vi "Tiling second try.vi"() -> ()   [LabVIEW 2020]
uses:
  <vilib>/DAQmx/write.llb/DAQmx Write (Analog 1D Wfm NChan NSamp).vi
  <vilib>/DAQmx/create/channels.llb/DAQmx Create Channel (AO-Voltage-Basic).vi
  <vilib>/DAQmx/configure/timing.llb/DAQmx Timing (Use Waveform).vi
  <vilib>/DAQmx/miscellaneous.llb/DAQmx Fill In Error Info.vi
  <vilib>/measure/NI_MABase.lvlib
panel:
  out "Y Position 4":dbl=3.1101367187499998
  in  "OK Button":bool
  in  "Sawtooth Amplitude":dbl=0.23 format="%.2p"
  in  "Sawtooth Phase":dbl=180.0 format="%.2p"
  in  "Stop Analog Signal":bool
  out "# Samples written per channel":u32=1000
  in  "Exposure time (ms)":dbl=1000.0
  in  "Camera trigger delay (degrees)":dbl=-10.0 format="%.2p"
  in  "Sawtooth Offset":dbl=0.008 format="%.2p"
  out "Waveform Graph":waveform(dbl)[](graph)=[{"t0"=timestamp(0 s since 1904-01-01), "dt"=0.001, "Y"=array[1000 elements]}, {"t0"=timestamp(0 s since 1904-01-01), "dt"=0.001, "Y"=array[1000 elements]}, {"t0"=timestamp(0 s since 1904-01-01), "dt"=0.001, "Y"=array[1000 elements]}]
  in  "Z step size (um)":dbl=-0.2
  out "Number of Slices":dbl=100.0
  in  "Input will be multiplied by 5":dbl=20.0
  out "Error out":errorcluster
  in  "Close Communication":bool
  out "Z Position":dbl=3.559384999999838
  out "GetFirmwareVersion 2":string="3.03\r"
  out "Connected":bool=TRUE
  in  "SPIIPLUSCOM660Lib.IAsyncChannel":refnum<k7>
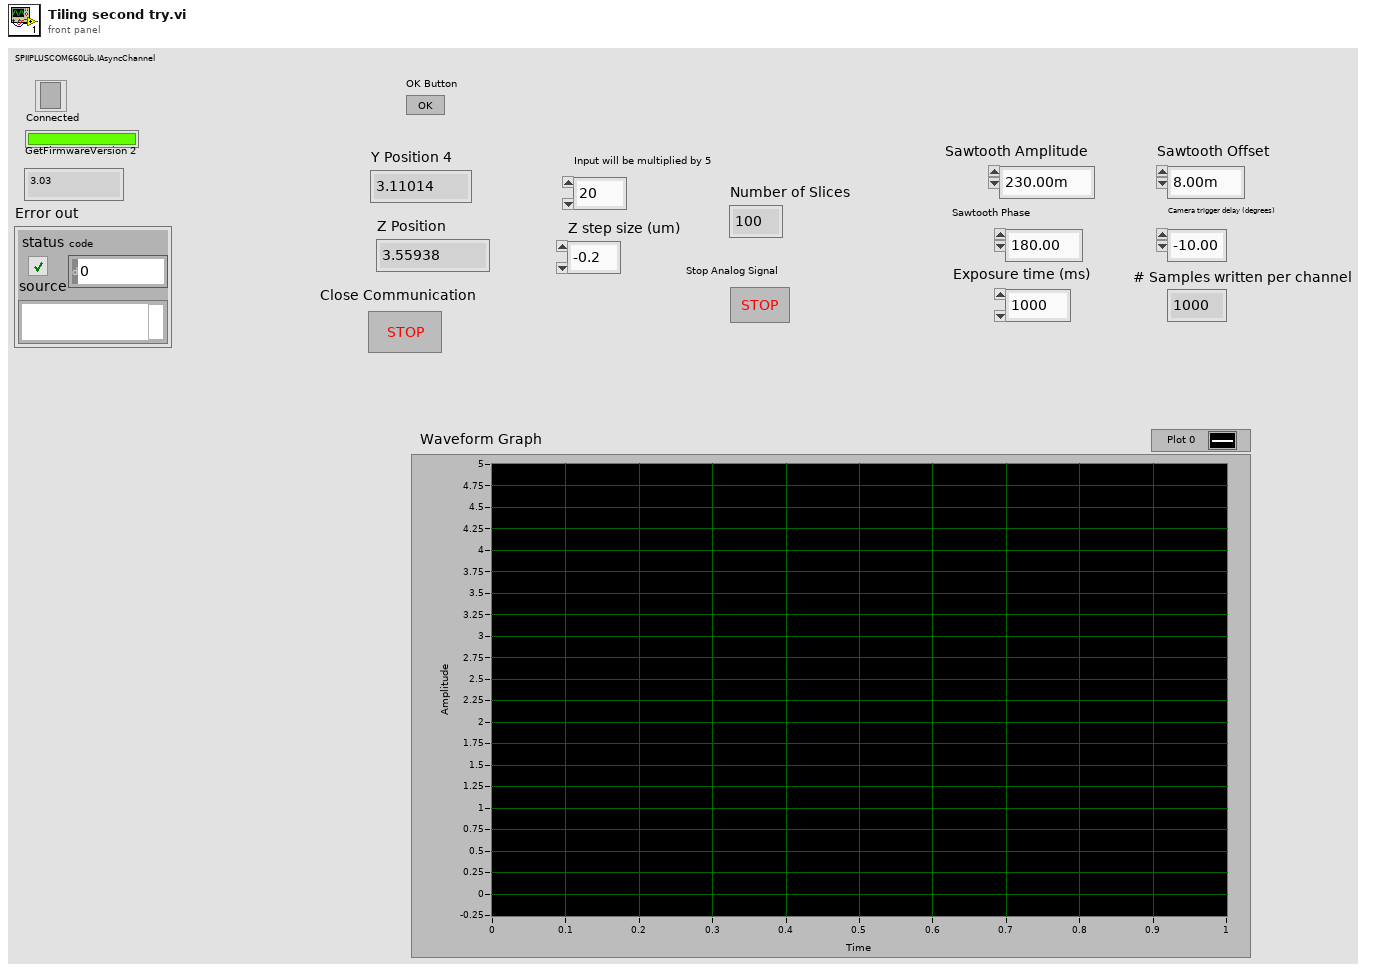
[diagram p1: front panel]
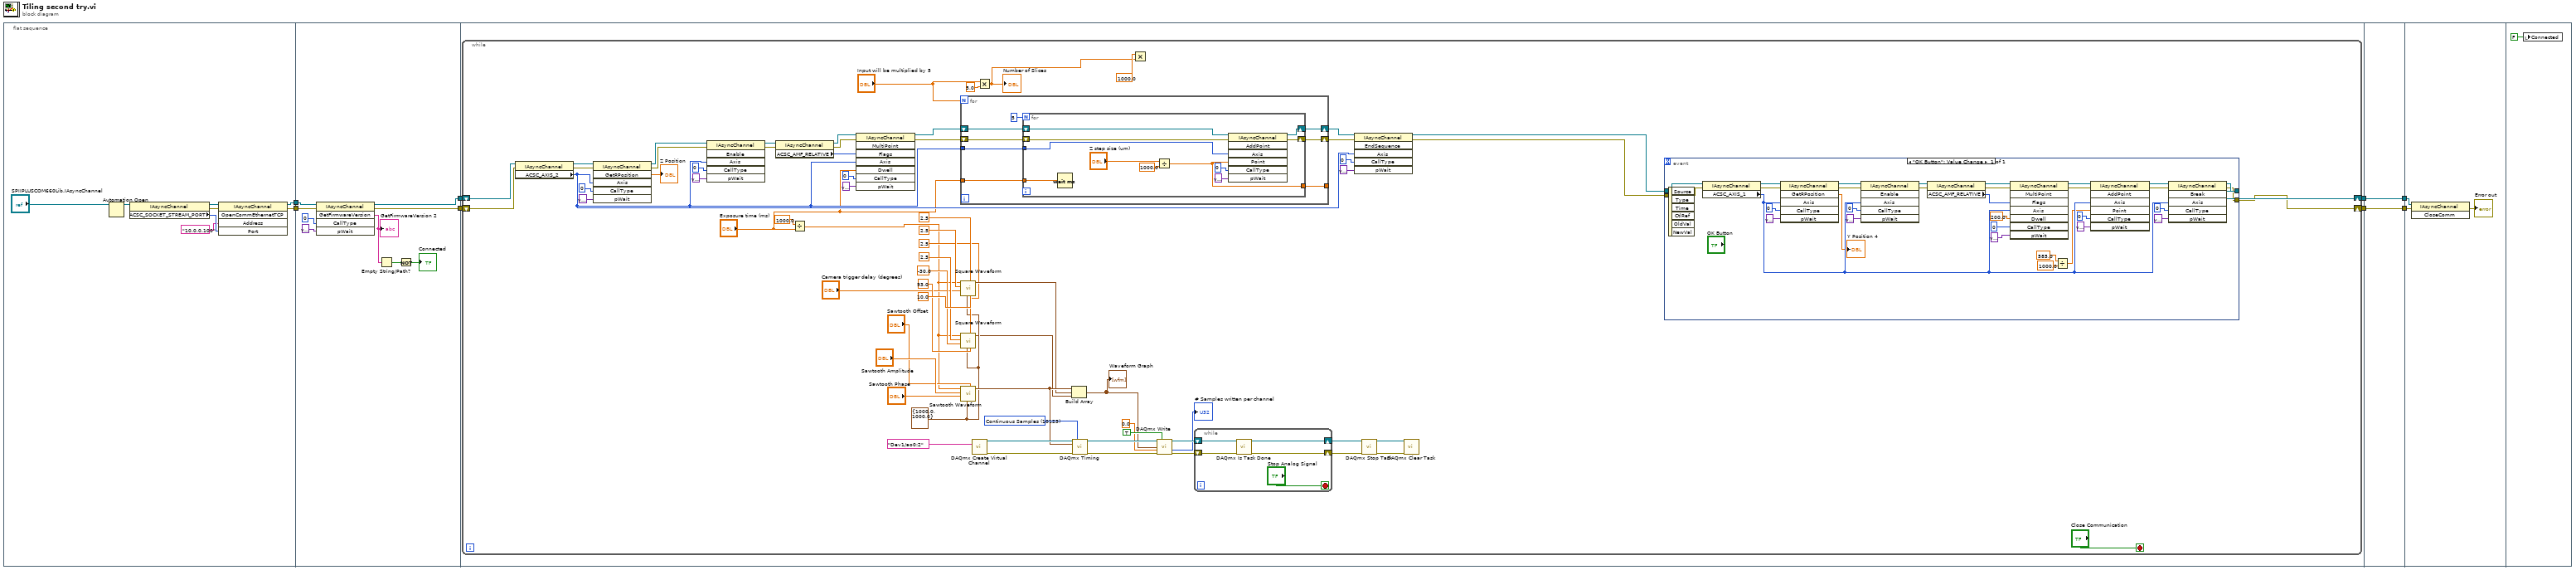
[diagram p0: block diagram]
diagram:
  n1 = flat-sequence {
    tunnel: [w11] -> w8
    tunnel: [w10] -> w7
    tunnel: w8 -> [w21]
    tunnel: w7 -> [w20]
    tunnel: [w18] -> w6
    tunnel: [w17] -> w5
    tunnel: w6 -> [w26]
    tunnel: w5 -> [w29]
    tunnel: [w28] -> w4
    tunnel: [w27] -> w3
    tunnel: w4 -> [w156]
    tunnel: w3 -> [w155]
    tunnel: [w156] -> w2
    tunnel: [w155] -> w1
    tunnel: w2 -> [w158]
    tunnel: w1 -> [w157]
    frame #0 {
      n2 = Automation Open(Automation Refnum="SPIIPLUSCOM660Lib.IAsyncChannel") -> (Automation Refnum=w16:refnum<k7>)  [unwired: 3 in, 1 out]
      n3 = property class="IAsyncChannel"(reference=w16) -> (reference out=w15:refnum<k7>, error out=w9:errorcluster, "ACSC_SOCKET_STREAM_PORT"=w13:i32)  [unwired: 1 in]
      n4 = invoke class="IAsyncChannel" method="OpenCommEthernetTCP"(reference=w15, error in=w9, "Address"="10.0.0.100", "Port"=w13) -> (reference out=w11:refnum<k7>, error out=w10:errorcluster)  [unwired: 1 in, 3 out]
    }
    frame #1 {
      n5 = invoke class="IAsyncChannel" method="GetFirmwareVersion"(reference=w21, error in=w20, "CallType"=u64 0, "pWait"=variant) -> (reference out=w18:refnum<k7>, error out=w17:errorcluster, "GetFirmwareVersion"=w23:string)  [unwired: 1 in, 2 out]
      "GetFirmwareVersion 2" <- w23
      n6 = Empty String/Path?(string/path=w23) -> (empty?=w22:bool)
      n7 = Not(x=w22) -> (.not. x?=→"Connected":bool)
    }
    frame #2 {
      n8 = while {
        shift-right: [w92] -> w28
        shift-left: w26 -> [w96]
        shift-right: [w91] -> w27
        shift-left: w29 -> [w95]
        stop <- "Close Communication" stop-if-true
        w54 = cluster{"Fs":dbl, "#s":dbl} {"Fs"=1000.0, "#s"=1000.0} ("sampling info")
        w77 = 10123 items=["Finite Samples"=10178, "Continuous Samples"=10123, "Hardware Timed Single Point"=12522] ("sample mode")
        n9 = property class="IAsyncChannel"(reference=w96, error in=w95) -> (reference out=w88:refnum<k7>, error out=w87:errorcluster, "ACSC_AXIS_2"=w90:i32)
        n10 = invoke class="IAsyncChannel" method="GetRPosition"(reference=w88, error in=w87, "Axis"=w90, "CallType"=u64 0, "pWait"=variant) -> (reference out=w36:refnum<k7>, error out=w34:errorcluster, "GetRPosition"=→"Z Position":dbl)  [unwired: 1 in, 3 out]
        n11 = invoke class="IAsyncChannel" method="Enable"(reference=w36, error in=w34, "Axis"=w90, "CallType"=u64 0, "pWait"=variant) -> (reference out=w35:refnum<k7>, error out=w33:errorcluster)  [unwired: 1 in, 4 out]
        n12 = property class="IAsyncChannel"(reference=w35, error in=w33) -> (reference out=w48:refnum<k7>, error out=w47:errorcluster, "ACSC_AMF_RELATIVE"=w44:i32)
        n13 = Divide(x=1000.0, y="Exposure time (ms)") -> (x/y=w53:dbl)
        n14 = invoke class="IAsyncChannel" method="MultiPoint"(reference=w48, error in=w47, "Flags"=w44, "Axis"=w90, "Dwell"="Exposure time (ms)", "CallType"=u64 0, "pWait"=variant) -> (reference out=w43:refnum<k7>, error out=w42:errorcluster)  [unwired: 1 in, 6 out]
        n15 = for {
          N: "Input will be multiplied by 5" -> [_]
          tunnel: w90 -> [w134]
          tunnel: "Exposure time (ms)" -> [w133]
          shift-right: [w136] -> w41
          shift-left: w43 -> [w138]
          shift-right: [w135] -> w40
          shift-left: w42 -> [w137]
          tunnel: [w131] -> _
          n16 = for {
            N: 5 -> [_]
            tunnel: w134 -> [w149]
            shift-right: [w144] -> w136
            shift-left: w138 -> [w148]
            shift-right: [w143] -> w135
            shift-left: w137 -> [w147]
            tunnel: w133 -> [w140]
            tunnel: [w139] -> w131
            n17 = Wait (ms)(milliseconds to wait=w140) -> ()  [unwired: 1 out]
            n18 = Divide(x="Z step size (um)", y=1000.0) -> (x/y=w139:dbl)
            n19 = invoke class="IAsyncChannel" method="AddPoint"(reference=w148, error in=w147, "Axis"=w149, "Point"=w139, "CallType"=u64 0, "pWait"=variant) -> (reference out=w144:refnum<k7>, error out=w143:errorcluster)  [unwired: 1 in, 5 out]
          }
        }
        n20 = call <vilib>:"Square Waveform.vi"("duty cycle (%)"=10.0, "offset"=2.5, "sampling info"=w54, "phase"="Camera trigger delay (degrees)", "amplitude"=2.5, "frequency"=w53) -> ("signal out"=w61:waveform(dbl))  [unwired: 4 in, 1 out]
        n21 = call <vilib>:"Square Waveform.vi"("duty cycle (%)"=93.0, "offset"=2.5, "sampling info"=w54, "phase"=-30.0, "amplitude"=2.5, "frequency"=w53) -> ("signal out"=w52:waveform(dbl))  [unwired: 4 in, 1 out]
        n22 = call <vilib>:"Sawtooth Waveform.vi"("offset"="Sawtooth Offset", "sampling info"=w54, "phase"="Sawtooth Phase", "amplitude"="Sawtooth Amplitude", "frequency"=w53) -> ("signal out"=w62:waveform(dbl))  [unwired: 5 in, 1 out]
        n23 = call-poly <vilib>:"DAQmx Create Virtual Channel.vi"("physical channels"=tag "Dev1/ao0:2") -> ("task out"=w79:refnum<k21>, "error out"=w78:errorcluster)  [unwired: 13 in]
        n24 = Multiply(x="Input will be multiplied by 5", y=5.0) -> (x*y=w30:dbl)
        "Number of Slices" <- w30
        n25 = Build Array(w62, w61, w52) -> (w51:waveform(dbl)[])
        "Waveform Graph" <- w51
        n26 = call-poly <vilib>:"DAQmx Timing.vi"("task/channels in"=w79, "sample mode"=w77, "waveform"=w62, "error in"=w78) -> ("task out"=w74:refnum<k21>, "error out"=w73:errorcluster)  [unwired: 10 in]
        n27 = Multiply(x=1000.0, y=w30) -> ()  [unwired: 1 out]
        n28 = call-poly <vilib>:"DAQmx Write.vi"("task/channels in"=w74, "auto start"=TRUE, "data"=w51, "timeout"=0.0, "error in"=w73) -> ("task out"=w75:refnum<k21>, "number of samples written per channel"=→"# Samples written per channel":u32, "error out"=w76:errorcluster)  [unwired: 8 in]
        n29 = while {
          shift-right: [w151] -> w70
          shift-left: w75 -> [w154]
          shift-right: [w152] -> w71
          shift-left: w76 -> [w153]
          stop <- "Stop Analog Signal" stop-if-true
          n30 = call <vilib>:"DAQmx Is Task Done.vi"("task/channels in"=w154, "error in"=w153) -> ("task out"=w151:refnum<k21>, "error out"=w152:errorcluster)  [unwired: 11 in, 1 out]
        }
        n31 = invoke class="IAsyncChannel" method="EndSequence"(reference=w41, error in=w40, "Axis"=w90, "CallType"=u64 0, "pWait"=variant) -> (reference out=w94:refnum<k7>, error out=w93:errorcluster)  [unwired: 1 in, 4 out]
        n32 = call <vilib>:"DAQmx Stop Task.vi"("task/channels in"=w70, "error in"=w71) -> ("task out"=w80:refnum<k21>, "error out"=w81:errorcluster)  [unwired: 12 in]
        n33 = call <vilib>:"DAQmx Clear Task.vi"("task in"=w80, "error in"=w81) -> ()  [unwired: 13 in, 1 out]
        n34 = event shown="[0] \"OK Button\": Value Change" {
          selector: _ -> [_]
          dyn-events: _ -> [_]
          timeout: _ -> [_]
          tunnel: w94 -> [w101]
          tunnel: w93 -> [w100]
          tunnel: [w99] -> w92
          tunnel: [w98] -> w91
          event "OK Button": Value Change {
            n35 = event-data() -> ()  [unwired: 1 in, 6 out]
            n36 = property class="IAsyncChannel"(reference=w101, error in=w100) -> (reference out=w123:refnum<k7>, error out=w124:errorcluster, "ACSC_AXIS_1"=w130:i32)
            n37 = invoke class="IAsyncChannel" method="GetRPosition"(reference=w123, error in=w124, "Axis"=w130, "CallType"=u64 0, "pWait"=variant) -> (reference out=w126:refnum<k7>, error out=w127:errorcluster, "GetRPosition"=→"Y Position 4":dbl)  [unwired: 1 in, 3 out]
            n38 = invoke class="IAsyncChannel" method="Enable"(reference=w126, error in=w127, "Axis"=w130, "CallType"=u64 0, "pWait"=variant) -> (reference out=w128:refnum<k7>, error out=w129:errorcluster)  [unwired: 1 in, 4 out]
            n39 = property class="IAsyncChannel"(reference=w128, error in=w129) -> (reference out=w115:refnum<k7>, error out=w116:errorcluster, "ACSC_AMF_RELATIVE"=w117:i32)
            n40 = invoke class="IAsyncChannel" method="MultiPoint"(reference=w115, error in=w116, "Flags"=w117, "Axis"=w130, "Dwell"=200.0, "CallType"=u64 0, "pWait"=variant) -> (reference out=w118:refnum<k7>, error out=w119:errorcluster)  [unwired: 1 in, 6 out]
            n41 = Divide(x=585.0, y=1000.0) -> (x/y=w122:dbl)
            n42 = invoke class="IAsyncChannel" method="AddPoint"(reference=w118, error in=w119, "Axis"=w130, "Point"=w122, "CallType"=u64 0, "pWait"=variant) -> (reference out=w120:refnum<k7>, error out=w121:errorcluster)  [unwired: 1 in, 5 out]
            n43 = invoke class="IAsyncChannel" method="Break"(reference=w120, error in=w121, "Axis"=w130, "CallType"=u64 0, "pWait"=variant) -> (reference out=w99:refnum<k7>, error out=w98:errorcluster)  [unwired: 1 in, 4 out]
          }
        }
      }
    }
    frame #3 {
    }
    frame #4 {
      n44 = invoke class="IAsyncChannel" method="CloseComm"(reference=w158, error in=w157) -> (error out=→"Error out":errorcluster)  [unwired: 1 in, 2 out]
    }
    frame #5 {
      n45 = local write "Connected"(FALSE ("Connected")) -> ()
    }
  }
